vi "BMU参数读取-Auto.vi"(7 "Socket":dbl, 8 "CAN端口":u16(ring), 9 "设备索引号":u16(ring), 10 "CAN卡类型":u32(ring)=21, 11 "从板号":u8=1) -> (3 "成功?":bool)   [LabVIEW 2013] (continued)
                n3264 = Select(t=0, s=w5020, f=1) -> (s? t:f=w5019:i32)
                n3265 = property on="电池组信息" class="Clust (严格)"("Disabled"=w5019) -> ()  [unwired: 2 in, 2 out]
                n3266 = property on="从板号" class="DigNum (严格)"("NumText.BGColor"=u32 16777215) -> ()  [unwired: 2 in, 2 out]
                n3267 = global read "功能码全局.vi" "24"() -> (w5016:bool[])
                n3268 = global read "功能码全局.vi" "23"() -> (w5017:bool[])
                n3269 = Index Array(array=w5016) -> (element #3=w5006:bool, element #4=w5005:bool, element #5=w5004:bool, element #6=w5003:bool, element #7=w5002:bool, element #8=w5001:bool)  [unwired: 8 in, 2 out]
                n3270 = Index Array(array=w5017) -> (element #3=w5015:bool, element #4=w5014:bool, element #5=w5013:bool, element #6=w5012:bool, element #7=w5011:bool, element #8=w5010:bool)  [unwired: 8 in, 2 out]
                n3271 = Build Array(w5006, w5005, w5004, w5003, w5002, w5001) -> (w5007:bool[])
                n3272 = Build Array(w5015, w5014, w5013, w5012, w5011, w5010) -> (w5009:bool[])
                n3273 = And Array Elements(Boolean array=w5007) -> (logical AND=w5000:bool)
                n3274 = And Array Elements(Boolean array=w5009) -> (logical AND=w5008:bool)
                n3275 = Not(x=w4999) -> (.not. x?=w5023:bool)
              }
              frame "电池包信息1" {
                w5028 = 2
                w5036 = 2
                w5027 = 2
                w5025 = FALSE ("1 6")
                n3276 = Select(t=0, s=w5033, f=1) -> (s? t:f=w5026:i32)
                n3277 = property on="串联数" class="DigNum (严格)"("Disabled"=w5026) -> ()  [unwired: 2 in, 2 out]
                n3278 = property on="并联数" class="DigNum (严格)"("Disabled"=w5026) -> ()  [unwired: 2 in, 2 out]
                n3279 = property on="电池厂家" class="DigNum (严格)"("Disabled"=w5026) -> ()  [unwired: 2 in, 2 out]
                n3280 = property on="电池类型" class="DigNum (严格)"("Disabled"=w5026) -> ()  [unwired: 2 in, 2 out]
                n3281 = property on="额定能量" class="DigNum (严格)"("Disabled"=w5026) -> ()  [unwired: 2 in, 2 out]
                n3282 = property on="额定容量" class="DigNum (严格)"("Disabled"=w5026) -> ()  [unwired: 2 in, 2 out]
                n3283 = property on="实际容量" class="DigNum (严格)"("Disabled"=w5026) -> ()  [unwired: 2 in, 2 out]
                n3284 = property on="电池组信息" class="Clust (严格)"("Disabled"=w5026) -> ()  [unwired: 2 in, 2 out]
                n3285 = property on="生产日期" class="Str"("DisabledEnum"=w5026) -> ()  [unwired: 2 in, 2 out]
                n3286 = property on="车牌号" class="Str"("DisabledEnum"=w5027) -> ()  [unwired: 2 in, 2 out]
                n3287 = property on="产权标识" class="DigNum (严格)"("Disabled"=w5026) -> ()  [unwired: 2 in, 2 out]
                n3288 = property on="应用车型" class="DigNum (严格)"("Disabled"=w5026) -> ()  [unwired: 2 in, 2 out]
                n3289 = property on="额定总压" class="DigNum (严格)"("Disabled"=w5026) -> ()  [unwired: 2 in, 2 out]
                n3290 = property on="电池包序号" class="DigNum (严格)"("DisabledEnum"=w5026) -> ()  [unwired: 2 in, 2 out]
                n3291 = property on="电池包组号" class="DigNum (严格)"("DisabledEnum"=w5027) -> ()  [unwired: 2 in, 2 out]
                n3292 = property on="最大允许单体电压" class="DigNum (严格)"("Disabled"=w5036) -> ()  [unwired: 2 in, 2 out]
                n3293 = property on="最大允许总电压" class="DigNum (严格)"("Disabled"=w5036) -> ()  [unwired: 2 in, 2 out]
                n3294 = property on="最大允许温度" class="DigNum (严格)"("Disabled"=w5036) -> ()  [unwired: 2 in, 2 out]
                n3295 = property on="最小允许温度" class="DigNum (严格)"("Disabled"=w5036) -> ()  [unwired: 2 in, 2 out]
                n3296 = property on="最大允许充电电流" class="DigNum (严格)"("Disabled"=w5036) -> ()  [unwired: 2 in, 2 out]
                n3297 = property on="最小允许充电电流" class="DigNum (严格)"("Disabled"=w5036) -> ()  [unwired: 2 in, 2 out]
                n3298 = property on="最小允许单体电压" class="DigNum (严格)"("Disabled"=w5036) -> ()  [unwired: 2 in, 2 out]
                n3299 = property on="电流步长" class="DigNum (严格)"("Disabled"=w5036) -> ()  [unwired: 2 in, 2 out]
                n3300 = property on="SOC" class="DigNum (严格)"("Disabled"=w5036) -> ()  [unwired: 2 in, 2 out]
                n3301 = property on="充电总安时" class="DigNum (严格)"("Disabled"=w5036) -> ()  [unwired: 2 in, 2 out]
                n3302 = property on="放电总安时" class="DigNum (严格)"("Disabled"=w5036) -> ()  [unwired: 2 in, 2 out]
                n3303 = property on="放空次数" class="DigNum (严格)"("DisabledEnum"=w5028) -> ()  [unwired: 2 in, 2 out]
                n3304 = property on="充满次数" class="DigNum (严格)"("DisabledEnum"=w5028) -> ()  [unwired: 2 in, 2 out]
                n3305 = property on="充电次数" class="DigNum (严格)"("DisabledEnum"=w5028) -> ()  [unwired: 2 in, 2 out]
                n3306 = global read "功能码全局.vi" "24"() -> (w5031:bool[])
                n3307 = global read "功能码全局.vi" "23"() -> (w5032:bool[])
                n3308 = Index Array(array=w5031) -> (element #3=w5029:bool)  [unwired: 8 in, 7 out]
                n3309 = Index Array(array=w5032) -> (element #3=w5030:bool)  [unwired: 8 in, 7 out]
                n3310 = Not(x=w5025) -> (.not. x?=w5037:bool)
              }
              frame "电池包组号" {
                w5042 = 2
                w5041 = 2
                w5051 = 2
                w5043 = 2
                w5052 = 2
                w5039 = FALSE ("1 6")
                n3311 = property on="串联数" class="DigNum (严格)"("Disabled"=w5052) -> ()  [unwired: 2 in, 2 out]
                n3312 = property on="并联数" class="DigNum (严格)"("Disabled"=w5052) -> ()  [unwired: 2 in, 2 out]
                n3313 = property on="电池厂家" class="DigNum (严格)"("Disabled"=w5052) -> ()  [unwired: 2 in, 2 out]
                n3314 = property on="电池类型" class="DigNum (严格)"("Disabled"=w5052) -> ()  [unwired: 2 in, 2 out]
                n3315 = property on="额定能量" class="DigNum (严格)"("Disabled"=w5052) -> ()  [unwired: 2 in, 2 out]
                n3316 = property on="额定容量" class="DigNum (严格)"("Disabled"=w5052) -> ()  [unwired: 2 in, 2 out]
                n3317 = property on="实际容量" class="DigNum (严格)"("Disabled"=w5052) -> ()  [unwired: 2 in, 2 out]
                n3318 = Select(t=0, s=w5048, f=1) -> (s? t:f=w5040:i32)
                n3319 = property on="生产日期" class="Str"("DisabledEnum"=w5042) -> ()  [unwired: 2 in, 2 out]
                n3320 = property on="电池包序号" class="DigNum (严格)"("DisabledEnum"=w5042) -> ()  [unwired: 2 in, 2 out]
                n3321 = property on="车牌号" class="Str"("DisabledEnum"=w5042) -> ()  [unwired: 2 in, 2 out]
                n3322 = property on="电池包组号" class="DigNum (严格)"("DisabledEnum"=w5040) -> ()  [unwired: 2 in, 2 out]
                n3323 = property on="电池组信息" class="Clust (严格)"("Disabled"=w5040) -> ()  [unwired: 2 in, 2 out]
                n3324 = property on="产权标识" class="DigNum (严格)"("Disabled"=w5043) -> ()  [unwired: 2 in, 2 out]
                n3325 = property on="应用车型" class="DigNum (严格)"("Disabled"=w5043) -> ()  [unwired: 2 in, 2 out]
                n3326 = property on="额定总压" class="DigNum (严格)"("Disabled"=w5043) -> ()  [unwired: 2 in, 2 out]
                n3327 = property on="放空次数" class="DigNum (严格)"("DisabledEnum"=w5041) -> ()  [unwired: 2 in, 2 out]
                n3328 = property on="充满次数" class="DigNum (严格)"("DisabledEnum"=w5041) -> ()  [unwired: 2 in, 2 out]
                n3329 = property on="充电次数" class="DigNum (严格)"("DisabledEnum"=w5041) -> ()  [unwired: 2 in, 2 out]
                n3330 = property on="最大允许单体电压" class="DigNum (严格)"("Disabled"=w5051) -> ()  [unwired: 2 in, 2 out]
                n3331 = property on="最大允许总电压" class="DigNum (严格)"("Disabled"=w5051) -> ()  [unwired: 2 in, 2 out]
                n3332 = property on="最大允许温度" class="DigNum (严格)"("Disabled"=w5051) -> ()  [unwired: 2 in, 2 out]
                n3333 = property on="最小允许温度" class="DigNum (严格)"("Disabled"=w5051) -> ()  [unwired: 2 in, 2 out]
                n3334 = property on="最大允许充电电流" class="DigNum (严格)"("Disabled"=w5051) -> ()  [unwired: 2 in, 2 out]
                n3335 = property on="最小允许充电电流" class="DigNum (严格)"("Disabled"=w5051) -> ()  [unwired: 2 in, 2 out]
                n3336 = property on="最小允许单体电压" class="DigNum (严格)"("Disabled"=w5051) -> ()  [unwired: 2 in, 2 out]
                n3337 = property on="电流步长" class="DigNum (严格)"("Disabled"=w5051) -> ()  [unwired: 2 in, 2 out]
                n3338 = property on="SOC" class="DigNum (严格)"("Disabled"=w5051) -> ()  [unwired: 2 in, 2 out]
                n3339 = property on="充电总安时" class="DigNum (严格)"("Disabled"=w5051) -> ()  [unwired: 2 in, 2 out]
                n3340 = property on="放电总安时" class="DigNum (严格)"("Disabled"=w5051) -> ()  [unwired: 2 in, 2 out]
                n3341 = global read "功能码全局.vi" "24"() -> (w5046:bool[])
                n3342 = global read "功能码全局.vi" "23"() -> (w5047:bool[])
                n3343 = Index Array(array=w5046) -> (element #3=w5044:bool)  [unwired: 8 in, 7 out]
                n3344 = Index Array(array=w5047) -> (element #3=w5045:bool)  [unwired: 8 in, 7 out]
                n3345 = Not(x=w5039) -> (.not. x?=w5053:bool)
              }
              frame "充放电安时" {
                w5057 = 2
                w5056 = 2
                w5066 = 2
                w5067 = 2
                w5069 = 2
                w5055 = FALSE ("1 6")
                n3346 = property on="串联数" class="DigNum (严格)"("Disabled"=w5069) -> ()  [unwired: 2 in, 2 out]
                n3347 = property on="并联数" class="DigNum (严格)"("Disabled"=w5069) -> ()  [unwired: 2 in, 2 out]
                n3348 = property on="电池厂家" class="DigNum (严格)"("Disabled"=w5069) -> ()  [unwired: 2 in, 2 out]
                n3349 = property on="电池类型" class="DigNum (严格)"("Disabled"=w5069) -> ()  [unwired: 2 in, 2 out]
                n3350 = property on="额定能量" class="DigNum (严格)"("Disabled"=w5069) -> ()  [unwired: 2 in, 2 out]
                n3351 = property on="额定容量" class="DigNum (严格)"("Disabled"=w5069) -> ()  [unwired: 2 in, 2 out]
                n3352 = property on="实际容量" class="DigNum (严格)"("Disabled"=w5069) -> ()  [unwired: 2 in, 2 out]
                n3353 = Select(t=0, s=w5063, f=1) -> (s? t:f=w5062:i32)
                n3354 = property on="生产日期" class="Str"("DisabledEnum"=w5057) -> ()  [unwired: 2 in, 2 out]
                n3355 = property on="电池包序号" class="DigNum (严格)"("DisabledEnum"=w5057) -> ()  [unwired: 2 in, 2 out]
                n3356 = property on="车牌号" class="Str"("DisabledEnum"=w5057) -> ()  [unwired: 2 in, 2 out]
                n3357 = property on="电池包组号" class="DigNum (严格)"("DisabledEnum"=w5057) -> ()  [unwired: 2 in, 2 out]
                n3358 = property on="电池组信息" class="Clust (严格)"("Disabled"=w5062) -> ()  [unwired: 2 in, 2 out]
                n3359 = property on="额定总压" class="DigNum (严格)"("Disabled"=2) -> ()  [unwired: 2 in, 2 out]
                n3360 = property on="产权标识" class="DigNum (严格)"("Disabled"=w5067) -> ()  [unwired: 2 in, 2 out]
                n3361 = property on="应用车型" class="DigNum (严格)"("Disabled"=w5067) -> ()  [unwired: 2 in, 2 out]
                n3362 = property on="放空次数" class="DigNum (严格)"("DisabledEnum"=w5056) -> ()  [unwired: 2 in, 2 out]
                n3363 = property on="充满次数" class="DigNum (严格)"("DisabledEnum"=w5056) -> ()  [unwired: 2 in, 2 out]
                n3364 = property on="充电次数" class="DigNum (严格)"("DisabledEnum"=w5056) -> ()  [unwired: 2 in, 2 out]
                n3365 = property on="最大允许单体电压" class="DigNum (严格)"("Disabled"=w5066) -> ()  [unwired: 2 in, 2 out]
                n3366 = property on="最大允许总电压" class="DigNum (严格)"("Disabled"=w5066) -> ()  [unwired: 2 in, 2 out]
                n3367 = property on="最大允许温度" class="DigNum (严格)"("Disabled"=w5066) -> ()  [unwired: 2 in, 2 out]
                n3368 = property on="最小允许温度" class="DigNum (严格)"("Disabled"=w5066) -> ()  [unwired: 2 in, 2 out]
                n3369 = property on="最大允许充电电流" class="DigNum (严格)"("Disabled"=w5066) -> ()  [unwired: 2 in, 2 out]
                n3370 = property on="最小允许充电电流" class="DigNum (严格)"("Disabled"=w5066) -> ()  [unwired: 2 in, 2 out]
                n3371 = property on="最小允许单体电压" class="DigNum (严格)"("Disabled"=w5066) -> ()  [unwired: 2 in, 2 out]
                n3372 = property on="电流步长" class="DigNum (严格)"("Disabled"=w5066) -> ()  [unwired: 2 in, 2 out]
                n3373 = property on="SOC" class="DigNum (严格)"("Disabled"=w5066) -> ()  [unwired: 2 in, 2 out]
                n3374 = property on="充电总安时" class="DigNum (严格)"("Disabled"=w5062) -> ()  [unwired: 2 in, 2 out]
                n3375 = property on="放电总安时" class="DigNum (严格)"("Disabled"=w5062) -> ()  [unwired: 2 in, 2 out]
                n3376 = Not(x=w5055) -> (.not. x?=w5070:bool)
                n3377 = global read "功能码全局.vi" "24"() -> (w5060:bool[])
                n3378 = global read "功能码全局.vi" "23"() -> (w5061:bool[])
                n3379 = Index Array(array=w5060) -> (element #7=w5058:bool)  [unwired: 8 in, 7 out]
                n3380 = Index Array(array=w5061) -> (element #7=w5059:bool)  [unwired: 8 in, 7 out]
              }
              frame "充电次数" {
                w5075 = 2
                w5084 = 2
                w5085 = 2
                w5076 = 2
                w5086 = 2
                w5072 = FALSE ("1 6")
                n3381 = property on="串联数" class="DigNum (严格)"("Disabled"=w5086) -> ()  [unwired: 2 in, 2 out]
                n3382 = property on="并联数" class="DigNum (严格)"("Disabled"=w5086) -> ()  [unwired: 2 in, 2 out]
                n3383 = property on="电池厂家" class="DigNum (严格)"("Disabled"=w5086) -> ()  [unwired: 2 in, 2 out]
                n3384 = property on="电池类型" class="DigNum (严格)"("Disabled"=w5086) -> ()  [unwired: 2 in, 2 out]
                n3385 = property on="额定能量" class="DigNum (严格)"("Disabled"=w5086) -> ()  [unwired: 2 in, 2 out]
                n3386 = property on="额定容量" class="DigNum (严格)"("Disabled"=w5086) -> ()  [unwired: 2 in, 2 out]
                n3387 = property on="实际容量" class="DigNum (严格)"("Disabled"=w5086) -> ()  [unwired: 2 in, 2 out]
                n3388 = Select(t=0, s=w5081, f=1) -> (s? t:f=w5073:i32)
                n3389 = property on="生产日期" class="Str"("DisabledEnum"=w5075) -> ()  [unwired: 2 in, 2 out]
                n3390 = property on="电池包序号" class="DigNum (严格)"("DisabledEnum"=w5075) -> ()  [unwired: 2 in, 2 out]
                n3391 = property on="车牌号" class="Str"("DisabledEnum"=w5075) -> ()  [unwired: 2 in, 2 out]
                n3392 = property on="电池组信息" class="Clust (严格)"("Disabled"=w5073) -> ()  [unwired: 2 in, 2 out]
                n3393 = property on="电池包组号" class="DigNum (严格)"("DisabledEnum"=w5075) -> ()  [unwired: 2 in, 2 out]
                n3394 = property on="额定总压" class="DigNum (严格)"("Disabled"=w5076) -> ()  [unwired: 2 in, 2 out]
                n3395 = property on="产权标识" class="DigNum (严格)"("Disabled"=w5076) -> ()  [unwired: 2 in, 2 out]
                n3396 = property on="应用车型" class="DigNum (严格)"("Disabled"=w5076) -> ()  [unwired: 2 in, 2 out]
                n3397 = property on="放空次数" class="DigNum (严格)"("DisabledEnum"=w5073) -> (error out=w5074:errorcluster)  [unwired: 2 in, 1 out]
                n3398 = property on="充满次数" class="DigNum (严格)"("DisabledEnum"=w5073) -> ()  [unwired: 2 in, 2 out]
                n3399 = property on="充电次数" class="DigNum (严格)"("DisabledEnum"=w5073) -> ()  [unwired: 2 in, 2 out]
                n3400 = property on="最大允许单体电压" class="DigNum (严格)"("Disabled"=w5085) -> ()  [unwired: 2 in, 2 out]
                n3401 = property on="最大允许总电压" class="DigNum (严格)"("Disabled"=w5085) -> ()  [unwired: 2 in, 2 out]
                n3402 = property on="最大允许温度" class="DigNum (严格)"("Disabled"=w5085) -> ()  [unwired: 2 in, 2 out]
                n3403 = property on="最小允许温度" class="DigNum (严格)"("Disabled"=w5085) -> ()  [unwired: 2 in, 2 out]
                n3404 = property on="最大允许充电电流" class="DigNum (严格)"("Disabled"=w5085) -> ()  [unwired: 2 in, 2 out]
                n3405 = property on="最小允许充电电流" class="DigNum (严格)"(error in=w5074, "Disabled"=w5085) -> ()  [unwired: 1 in, 2 out]
                n3406 = property on="最小允许单体电压" class="DigNum (严格)"("Disabled"=w5085) -> ()  [unwired: 2 in, 2 out]
                n3407 = property on="电流步长" class="DigNum (严格)"("Disabled"=w5085) -> ()  [unwired: 2 in, 2 out]
                n3408 = property on="SOC" class="DigNum (严格)"("Disabled"=w5085) -> ()  [unwired: 2 in, 2 out]
                n3409 = property on="充电总安时" class="DigNum (严格)"("Disabled"=w5084) -> ()  [unwired: 2 in, 2 out]
                n3410 = property on="放电总安时" class="DigNum (严格)"("Disabled"=w5084) -> ()  [unwired: 2 in, 2 out]
                n3411 = Not(x=w5072) -> (.not. x?=w5087:bool)
                n3412 = global read "功能码全局.vi" "24"() -> (w5079:bool[])
                n3413 = global read "功能码全局.vi" "23"() -> (w5080:bool[])
                n3414 = Index Array(array=w5079) -> (element #8=w5078:bool)  [unwired: 8 in, 7 out]
                n3415 = Index Array(array=w5080) -> (element #8=w5077:bool)  [unwired: 8 in, 7 out]
              }
              frame "SOC" {
                w5091 = 2
                w5090 = 2
                w5100 = 2
                w5101 = 2
                w5102 = 2
                w5104 = 2
                w5089 = FALSE ("1 6")
                n3416 = property on="串联数" class="DigNum (严格)"("Disabled"=w5104) -> ()  [unwired: 2 in, 2 out]
                n3417 = property on="并联数" class="DigNum (严格)"("Disabled"=w5104) -> ()  [unwired: 2 in, 2 out]
                n3418 = property on="电池厂家" class="DigNum (严格)"("Disabled"=w5104) -> ()  [unwired: 2 in, 2 out]
                n3419 = property on="电池类型" class="DigNum (严格)"("Disabled"=w5104) -> ()  [unwired: 2 in, 2 out]
                n3420 = property on="额定能量" class="DigNum (严格)"("Disabled"=w5104) -> ()  [unwired: 2 in, 2 out]
                n3421 = property on="额定容量" class="DigNum (严格)"("Disabled"=w5104) -> ()  [unwired: 2 in, 2 out]
                n3422 = property on="实际容量" class="DigNum (严格)"("Disabled"=w5104) -> ()  [unwired: 2 in, 2 out]
                n3423 = Select(t=0, s=w5097, f=1) -> (s? t:f=w5096:i32)
                n3424 = property on="生产日期" class="Str"("DisabledEnum"=w5091) -> ()  [unwired: 2 in, 2 out]
                n3425 = property on="电池包序号" class="DigNum (严格)"("DisabledEnum"=w5091) -> ()  [unwired: 2 in, 2 out]
                n3426 = property on="车牌号" class="Str"("DisabledEnum"=w5091) -> ()  [unwired: 2 in, 2 out]
                n3427 = property on="电池包组号" class="DigNum (严格)"("DisabledEnum"=w5091) -> ()  [unwired: 2 in, 2 out]
                n3428 = property on="电池组信息" class="Clust (严格)"("Disabled"=w5096) -> ()  [unwired: 2 in, 2 out]
                n3429 = property on="SOC" class="DigNum (严格)"("Disabled"=w5096) -> ()  [unwired: 2 in, 2 out]
                n3430 = property on="额定总压" class="DigNum (严格)"("Disabled"=2) -> ()  [unwired: 2 in, 2 out]
                n3431 = property on="产权标识" class="DigNum (严格)"("Disabled"=w5102) -> ()  [unwired: 2 in, 2 out]
                n3432 = property on="应用车型" class="DigNum (严格)"("Disabled"=w5102) -> ()  [unwired: 2 in, 2 out]
                n3433 = property on="放空次数" class="DigNum (严格)"("DisabledEnum"=w5090) -> ()  [unwired: 2 in, 2 out]
                n3434 = property on="充满次数" class="DigNum (严格)"("DisabledEnum"=w5090) -> ()  [unwired: 2 in, 2 out]
                n3435 = property on="充电次数" class="DigNum (严格)"("DisabledEnum"=w5090) -> ()  [unwired: 2 in, 2 out]
                n3436 = property on="最大允许单体电压" class="DigNum (严格)"("Disabled"=w5101) -> ()  [unwired: 2 in, 2 out]
                n3437 = property on="最大允许总电压" class="DigNum (严格)"("Disabled"=w5101) -> ()  [unwired: 2 in, 2 out]
                n3438 = property on="最大允许温度" class="DigNum (严格)"("Disabled"=w5101) -> ()  [unwired: 2 in, 2 out]
                n3439 = property on="最小允许温度" class="DigNum (严格)"("Disabled"=w5101) -> ()  [unwired: 2 in, 2 out]
                n3440 = property on="最大允许充电电流" class="DigNum (严格)"("Disabled"=w5101) -> ()  [unwired: 2 in, 2 out]
                n3441 = property on="最小允许充电电流" class="DigNum (严格)"("Disabled"=w5101) -> ()  [unwired: 2 in, 2 out]
                n3442 = property on="最小允许单体电压" class="DigNum (严格)"("Disabled"=w5101) -> ()  [unwired: 2 in, 2 out]
                n3443 = property on="电流步长" class="DigNum (严格)"("Disabled"=w5101) -> ()  [unwired: 2 in, 2 out]
                n3444 = property on="充电总安时" class="DigNum (严格)"("Disabled"=w5100) -> ()  [unwired: 2 in, 2 out]
                n3445 = property on="放电总安时" class="DigNum (严格)"("Disabled"=w5100) -> ()  [unwired: 2 in, 2 out]
                n3446 = Not(x=w5089) -> (.not. x?=w5105:bool)
                n3447 = global read "功能码全局.vi" "24"() -> (w5094:bool[])
                n3448 = global read "功能码全局.vi" "23"() -> (w5095:bool[])
                n3449 = Index Array(array=w5094) -> (element #6=w5093:bool)  [unwired: 8 in, 7 out]
                n3450 = Index Array(array=w5095) -> (element #6=w5092:bool)  [unwired: 8 in, 7 out]
              }
              frame "车牌号" {
                w5110 = 2
                w5109 = 2
                w5119 = 2
                w5120 = 2
                w5121 = 2
                w5123 = 2
                w5107 = FALSE ("1 6")
                n3451 = property on="串联数" class="DigNum (严格)"("Disabled"=w5123) -> ()  [unwired: 2 in, 2 out]
                n3452 = property on="并联数" class="DigNum (严格)"("Disabled"=w5123) -> ()  [unwired: 2 in, 2 out]
                n3453 = property on="电池厂家" class="DigNum (严格)"("Disabled"=w5123) -> ()  [unwired: 2 in, 2 out]
                n3454 = property on="电池类型" class="DigNum (严格)"("Disabled"=w5123) -> ()  [unwired: 2 in, 2 out]
                n3455 = property on="额定能量" class="DigNum (严格)"("Disabled"=w5123) -> ()  [unwired: 2 in, 2 out]
                n3456 = property on="额定容量" class="DigNum (严格)"("Disabled"=w5123) -> ()  [unwired: 2 in, 2 out]
                n3457 = property on="实际容量" class="DigNum (严格)"("Disabled"=w5123) -> ()  [unwired: 2 in, 2 out]
                n3458 = Select(t=0, s=w5115, f=1) -> (s? t:f=w5108:i32)
                n3459 = property on="生产日期" class="Str"("DisabledEnum"=w5110) -> ()  [unwired: 2 in, 2 out]
                n3460 = property on="电池包序号" class="DigNum (严格)"("DisabledEnum"=w5110) -> ()  [unwired: 2 in, 2 out]
                n3461 = property on="电池包组号" class="DigNum (严格)"("DisabledEnum"=w5110) -> ()  [unwired: 2 in, 2 out]
                n3462 = property on="电池组信息" class="Clust (严格)"("Disabled"=w5108) -> ()  [unwired: 2 in, 2 out]
                n3463 = property on="车牌号" class="Str"("DisabledEnum"=w5108) -> ()  [unwired: 2 in, 2 out]
                n3464 = property on="额定总压" class="DigNum (严格)"("Disabled"=2) -> ()  [unwired: 2 in, 2 out]
                n3465 = property on="产权标识" class="DigNum (严格)"("Disabled"=w5121) -> ()  [unwired: 2 in, 2 out]
                n3466 = property on="应用车型" class="DigNum (严格)"("Disabled"=w5121) -> ()  [unwired: 2 in, 2 out]
                n3467 = property on="放空次数" class="DigNum (严格)"("DisabledEnum"=w5109) -> ()  [unwired: 2 in, 2 out]
                n3468 = property on="充满次数" class="DigNum (严格)"("DisabledEnum"=w5109) -> ()  [unwired: 2 in, 2 out]
                n3469 = property on="充电次数" class="DigNum (严格)"("DisabledEnum"=w5109) -> ()  [unwired: 2 in, 2 out]
                n3470 = property on="最大允许单体电压" class="DigNum (严格)"("Disabled"=w5120) -> ()  [unwired: 2 in, 2 out]
                n3471 = property on="最大允许总电压" class="DigNum (严格)"("Disabled"=w5120) -> ()  [unwired: 2 in, 2 out]
                n3472 = property on="最大允许温度" class="DigNum (严格)"("Disabled"=w5120) -> ()  [unwired: 2 in, 2 out]
                n3473 = property on="最小允许温度" class="DigNum (严格)"("Disabled"=w5120) -> ()  [unwired: 2 in, 2 out]
                n3474 = property on="最大允许充电电流" class="DigNum (严格)"("Disabled"=w5120) -> ()  [unwired: 2 in, 2 out]
                n3475 = property on="最小允许充电电流" class="DigNum (严格)"("Disabled"=w5120) -> ()  [unwired: 2 in, 2 out]
                n3476 = property on="最小允许单体电压" class="DigNum (严格)"("Disabled"=w5120) -> ()  [unwired: 2 in, 2 out]
                n3477 = property on="电流步长" class="DigNum (严格)"("Disabled"=w5120) -> ()  [unwired: 2 in, 2 out]
                n3478 = property on="SOC" class="DigNum (严格)"("Disabled"=2) -> ()  [unwired: 2 in, 2 out]
                n3479 = property on="充电总安时" class="DigNum (严格)"("Disabled"=w5119) -> ()  [unwired: 2 in, 2 out]
                n3480 = property on="放电总安时" class="DigNum (严格)"("Disabled"=w5119) -> ()  [unwired: 2 in, 2 out]
                n3481 = Not(x=w5107) -> (.not. x?=w5124:bool)
                n3482 = global read "功能码全局.vi" "24"() -> (w5113:bool[])
                n3483 = global read "功能码全局.vi" "23"() -> (w5114:bool[])
                n3484 = Index Array(array=w5113) -> (element #5=w5111:bool)  [unwired: 8 in, 7 out]
                n3485 = Index Array(array=w5114) -> (element #5=w5112:bool)  [unwired: 8 in, 7 out]
              }
              frame "充电参数" {
                w5128 = 2
                w5127 = 2
                w5137 = 2
                w5138 = 2
                w5140 = 2
                w5126 = FALSE ("1 6")
                n3486 = property on="串联数" class="DigNum (严格)"("Disabled"=w5140) -> ()  [unwired: 2 in, 2 out]
                n3487 = property on="并联数" class="DigNum (严格)"("Disabled"=w5140) -> ()  [unwired: 2 in, 2 out]
                n3488 = property on="电池厂家" class="DigNum (严格)"("Disabled"=w5140) -> ()  [unwired: 2 in, 2 out]
                n3489 = property on="电池类型" class="DigNum (严格)"("Disabled"=w5140) -> ()  [unwired: 2 in, 2 out]
                n3490 = property on="额定能量" class="DigNum (严格)"("Disabled"=w5140) -> ()  [unwired: 2 in, 2 out]
                n3491 = property on="额定容量" class="DigNum (严格)"("Disabled"=w5140) -> ()  [unwired: 2 in, 2 out]
                n3492 = property on="实际容量" class="DigNum (严格)"("Disabled"=w5140) -> ()  [unwired: 2 in, 2 out]
                n3493 = Select(t=0, s=w5134, f=1) -> (s? t:f=w5133:i32)
                n3494 = property on="生产日期" class="Str"("DisabledEnum"=w5128) -> ()  [unwired: 2 in, 2 out]
                n3495 = property on="电池包序号" class="DigNum (严格)"("DisabledEnum"=w5128) -> ()  [unwired: 2 in, 2 out]
                n3496 = property on="车牌号" class="Str"("DisabledEnum"=w5128) -> ()  [unwired: 2 in, 2 out]
                n3497 = property on="电池组信息" class="Clust (严格)"("Disabled"=w5133) -> ()  [unwired: 2 in, 2 out]
                n3498 = property on="电池包组号" class="DigNum (严格)"("DisabledEnum"=w5128) -> ()  [unwired: 2 in, 2 out]
                n3499 = property on="额定总压" class="DigNum (严格)"("Disabled"=2) -> ()  [unwired: 2 in, 2 out]
                n3500 = property on="产权标识" class="DigNum (严格)"("Disabled"=w5138) -> ()  [unwired: 2 in, 2 out]
                n3501 = property on="应用车型" class="DigNum (严格)"("Disabled"=w5138) -> ()  [unwired: 2 in, 2 out]
                n3502 = property on="放空次数" class="DigNum (严格)"("DisabledEnum"=w5127) -> ()  [unwired: 2 in, 2 out]
                n3503 = property on="充满次数" class="DigNum (严格)"("DisabledEnum"=w5127) -> ()  [unwired: 2 in, 2 out]
                n3504 = property on="充电次数" class="DigNum (严格)"("DisabledEnum"=w5127) -> ()  [unwired: 2 in, 2 out]
                n3505 = property on="最大允许单体电压" class="DigNum (严格)"("Disabled"=w5133) -> ()  [unwired: 2 in, 2 out]
                n3506 = property on="最大允许总电压" class="DigNum (严格)"("Disabled"=w5133) -> ()  [unwired: 2 in, 2 out]
                n3507 = property on="最大允许温度" class="DigNum (严格)"("Disabled"=w5133) -> ()  [unwired: 2 in, 2 out]
                n3508 = property on="最小允许温度" class="DigNum (严格)"("Disabled"=w5133) -> ()  [unwired: 2 in, 2 out]
                n3509 = property on="最大允许充电电流" class="DigNum (严格)"("Disabled"=w5133) -> ()  [unwired: 2 in, 2 out]
                n3510 = property on="最小允许充电电流" class="DigNum (严格)"("Disabled"=w5133) -> ()  [unwired: 2 in, 2 out]
                n3511 = property on="最小允许单体电压" class="DigNum (严格)"("Disabled"=w5133) -> ()  [unwired: 2 in, 2 out]
                n3512 = property on="电流步长" class="DigNum (严格)"("Disabled"=w5133) -> ()  [unwired: 2 in, 2 out]
                n3513 = property on="SOC" class="DigNum (严格)"("Disabled"=w5137) -> ()  [unwired: 2 in, 2 out]
                n3514 = property on="充电总安时" class="DigNum (严格)"("Disabled"=w5137) -> ()  [unwired: 2 in, 2 out]
                n3515 = property on="放电总安时" class="DigNum (严格)"("Disabled"=w5137) -> ()  [unwired: 2 in, 2 out]
                n3516 = Not(x=w5126) -> (.not. x?=w5141:bool)
                n3517 = global read "功能码全局.vi" "24"() -> (w5131:bool[])
                n3518 = global read "功能码全局.vi" "23"() -> (w5132:bool[])
                n3519 = Index Array(array=w5131) -> (element #4=w5129:bool)  [unwired: 8 in, 7 out]
                n3520 = Index Array(array=w5132) -> (element #4=w5130:bool)  [unwired: 8 in, 7 out]
              }
              frame "均衡参数" {
                w5143 = FALSE ("1 6")
                n3521 = Select(t=0, s=w5149, f=1) -> (s? t:f=w5147:i32)
                n3522 = property on="均衡计算-电压高阀值1级" class="DigNum (严格)"("DisabledEnum"=w5147) -> ()  [unwired: 2 in, 2 out]
                n3523 = property on="均衡计算-电压高阀值2级" class="DigNum (严格)"("DisabledEnum"=w5147) -> ()  [unwired: 2 in, 2 out]
                n3524 = property on="均衡计算-电压低阀值1级" class="DigNum (严格)"("DisabledEnum"=w5147) -> ()  [unwired: 2 in, 2 out]
                n3525 = property on="均衡计算-电压低阀值2级" class="DigNum (严格)"("DisabledEnum"=w5147) -> ()  [unwired: 2 in, 2 out]
                n3526 = property on="均衡计算-最低电压阀值" class="DigNum (严格)"("DisabledEnum"=w5147) -> ()  [unwired: 2 in, 2 out]
                n3527 = property on="均衡停止-最低电压阀值" class="DigNum (严格)"("DisabledEnum"=w5147) -> ()  [unwired: 2 in, 2 out]
                n3528 = property on="均衡计算-电压极差阀值" class="DigNum (严格)"("DisabledEnum"=w5147) -> ()  [unwired: 2 in, 2 out]
                n3529 = property on="均衡参数" class="Clust (严格)"("DisabledEnum"=w5147) -> ()  [unwired: 2 in, 2 out]
                n3530 = property on="充电结束电压(90%)" class="DigNum (严格)"("DisabledEnum"=w5147) -> ()  [unwired: 2 in, 2 out]
                n3531 = property on="充电结束电压(91%)" class="DigNum (严格)"("DisabledEnum"=w5147) -> ()  [unwired: 2 in, 2 out]
                n3532 = property on="充电结束电压(92%)" class="DigNum (严格)"("DisabledEnum"=w5147) -> ()  [unwired: 2 in, 2 out]
                n3533 = property on="充电结束电压(93%)" class="DigNum (严格)"("DisabledEnum"=w5147) -> ()  [unwired: 2 in, 2 out]
                n3534 = property on="充电结束电压(94%)" class="DigNum (严格)"("DisabledEnum"=w5147) -> ()  [unwired: 2 in, 2 out]
                n3535 = property on="充电结束电压(95%)" class="DigNum (严格)"("DisabledEnum"=w5147) -> ()  [unwired: 2 in, 2 out]
                n3536 = property on="充电结束电压(96%)" class="DigNum (严格)"("DisabledEnum"=w5147) -> ()  [unwired: 2 in, 2 out]
                n3537 = property on="充电结束电压(97%)" class="DigNum (严格)"("DisabledEnum"=w5147) -> ()  [unwired: 2 in, 2 out]
                n3538 = property on="充电结束电压(98%)" class="DigNum (严格)"("DisabledEnum"=w5147) -> ()  [unwired: 2 in, 2 out]
                n3539 = property on="充电结束电压(99%)" class="DigNum (严格)"("DisabledEnum"=w5147) -> ()  [unwired: 2 in, 2 out]
                n3540 = property on="充电结束电压(100%)" class="DigNum (严格)"("DisabledEnum"=w5147) -> ()  [unwired: 2 in, 2 out]
                n3541 = disable-structure shown="启用" {
                  disable-tunnel: [w5153 w5155] -> w5146
                  disable-tunnel: [w5152 w5155] -> w5145
                  frame Enabled {
                    n3542 = global read "功能码全局.vi" "18"() -> (w5154:bool[])
                    n3543 = Index Array(array=w5154) -> (element #1=w5153:bool, element #2=w5152:bool)  [unwired: 8 in, 6 out]
                  }
                  frame Disabled {
                    w5155 = TRUE
                  }
                }
                n3544 = Not(x=w5143) -> (.not. x?=w5144:bool)
              }
              frame "均衡阀值" {
                w5158 = 2
                w5156 = FALSE ("1 6")
                n3545 = Select(t=0, s=w5163, f=1) -> (s? t:f=w5161:i32)
                n3546 = property on="均衡计算-电压高阀值1级" class="DigNum (严格)"("DisabledEnum"=w5161) -> ()  [unwired: 2 in, 2 out]
                n3547 = property on="均衡计算-电压高阀值2级" class="DigNum (严格)"("DisabledEnum"=w5161) -> ()  [unwired: 2 in, 2 out]
                n3548 = property on="均衡计算-电压低阀值1级" class="DigNum (严格)"("DisabledEnum"=w5161) -> ()  [unwired: 2 in, 2 out]
                n3549 = property on="均衡计算-电压低阀值2级" class="DigNum (严格)"("DisabledEnum"=w5161) -> ()  [unwired: 2 in, 2 out]
                n3550 = property on="均衡计算-最低电压阀值" class="DigNum (严格)"("DisabledEnum"=w5161) -> ()  [unwired: 2 in, 2 out]
                n3551 = property on="均衡停止-最低电压阀值" class="DigNum (严格)"("DisabledEnum"=w5161) -> ()  [unwired: 2 in, 2 out]
                n3552 = property on="均衡计算-电压极差阀值" class="DigNum (严格)"("DisabledEnum"=w5161) -> ()  [unwired: 2 in, 2 out]
                n3553 = property on="均衡参数" class="Clust (严格)"("DisabledEnum"=w5161) -> ()  [unwired: 2 in, 2 out]
                n3554 = property on="充电结束电压(90%)" class="DigNum (严格)"("DisabledEnum"=w5158) -> ()  [unwired: 2 in, 2 out]
                n3555 = property on="充电结束电压(91%)" class="DigNum (严格)"("DisabledEnum"=w5158) -> ()  [unwired: 2 in, 2 out]
                n3556 = property on="充电结束电压(92%)" class="DigNum (严格)"("DisabledEnum"=w5158) -> ()  [unwired: 2 in, 2 out]
                n3557 = property on="充电结束电压(93%)" class="DigNum (严格)"("DisabledEnum"=w5158) -> ()  [unwired: 2 in, 2 out]
                n3558 = property on="充电结束电压(94%)" class="DigNum (严格)"("DisabledEnum"=w5158) -> ()  [unwired: 2 in, 2 out]
                n3559 = property on="充电结束电压(95%)" class="DigNum (严格)"("DisabledEnum"=w5158) -> ()  [unwired: 2 in, 2 out]
                n3560 = property on="充电结束电压(96%)" class="DigNum (严格)"("DisabledEnum"=w5158) -> ()  [unwired: 2 in, 2 out]
                n3561 = property on="充电结束电压(97%)" class="DigNum (严格)"("DisabledEnum"=w5158) -> ()  [unwired: 2 in, 2 out]
                n3562 = property on="充电结束电压(98%)" class="DigNum (严格)"("DisabledEnum"=w5158) -> ()  [unwired: 2 in, 2 out]
                n3563 = property on="充电结束电压(99%)" class="DigNum (严格)"("DisabledEnum"=w5158) -> ()  [unwired: 2 in, 2 out]
                n3564 = property on="充电结束电压(100%)" class="DigNum (严格)"("DisabledEnum"=w5158) -> ()  [unwired: 2 in, 2 out]
                n3565 = disable-structure shown="启用" {
                  disable-tunnel: [w5167 w5169] -> w5160
                  disable-tunnel: [w5166 w5169] -> w5159
                  frame Enabled {
                    n3566 = global read "功能码全局.vi" "18"() -> (w5168:bool[])
                    n3567 = Index Array(array=w5168) -> (element #1=w5167:bool, element #2=w5166:bool)  [unwired: 8 in, 6 out]
                  }
                  frame Disabled {
                    w5169 = TRUE
                  }
                }
                n3568 = Not(x=w5156) -> (.not. x?=w5157:bool)
              }
              frame "充电结束电压" {
                w5173 = 2
                w5170 = FALSE ("1 6")
                n3569 = Select(t=0, s=w5177, f=1) -> (s? t:f=w5172:i32)
                n3570 = property on="均衡计算-电压高阀值1级" class="DigNum (严格)"("DisabledEnum"=w5173) -> ()  [unwired: 2 in, 2 out]
                n3571 = property on="均衡计算-电压高阀值2级" class="DigNum (严格)"("DisabledEnum"=w5173) -> ()  [unwired: 2 in, 2 out]
                n3572 = property on="均衡计算-电压低阀值1级" class="DigNum (严格)"("DisabledEnum"=w5173) -> ()  [unwired: 2 in, 2 out]
                n3573 = property on="均衡计算-电压低阀值2级" class="DigNum (严格)"("DisabledEnum"=w5173) -> ()  [unwired: 2 in, 2 out]
                n3574 = property on="均衡计算-最低电压阀值" class="DigNum (严格)"("DisabledEnum"=w5173) -> ()  [unwired: 2 in, 2 out]
                n3575 = property on="均衡停止-最低电压阀值" class="DigNum (严格)"("DisabledEnum"=w5173) -> ()  [unwired: 2 in, 2 out]
                n3576 = property on="均衡计算-电压极差阀值" class="DigNum (严格)"("DisabledEnum"=w5173) -> ()  [unwired: 2 in, 2 out]
                n3577 = property on="均衡参数" class="Clust (严格)"("DisabledEnum"=w5172) -> ()  [unwired: 2 in, 2 out]
                n3578 = property on="充电结束电压(90%)" class="DigNum (严格)"("DisabledEnum"=w5172) -> ()  [unwired: 2 in, 2 out]
                n3579 = property on="充电结束电压(91%)" class="DigNum (严格)"("DisabledEnum"=w5172) -> ()  [unwired: 2 in, 2 out]
                n3580 = property on="充电结束电压(92%)" class="DigNum (严格)"("DisabledEnum"=w5172) -> ()  [unwired: 2 in, 2 out]
                n3581 = property on="充电结束电压(93%)" class="DigNum (严格)"("DisabledEnum"=w5172) -> ()  [unwired: 2 in, 2 out]
                n3582 = property on="充电结束电压(94%)" class="DigNum (严格)"("DisabledEnum"=w5172) -> ()  [unwired: 2 in, 2 out]
                n3583 = property on="充电结束电压(95%)" class="DigNum (严格)"("DisabledEnum"=w5172) -> ()  [unwired: 2 in, 2 out]
                n3584 = property on="充电结束电压(96%)" class="DigNum (严格)"("DisabledEnum"=w5172) -> ()  [unwired: 2 in, 2 out]
                n3585 = property on="充电结束电压(97%)" class="DigNum (严格)"("DisabledEnum"=w5172) -> ()  [unwired: 2 in, 2 out]
                n3586 = property on="充电结束电压(98%)" class="DigNum (严格)"("DisabledEnum"=w5172) -> ()  [unwired: 2 in, 2 out]
                n3587 = property on="充电结束电压(99%)" class="DigNum (严格)"("DisabledEnum"=w5172) -> ()  [unwired: 2 in, 2 out]
                n3588 = property on="充电结束电压(100%)" class="DigNum (严格)"("DisabledEnum"=w5172) -> ()  [unwired: 2 in, 2 out]
                n3589 = disable-structure shown="启用" {
                  disable-tunnel: [w5181 w5183] -> w5175
                  disable-tunnel: [w5180 w5183] -> w5174
                  frame Enabled {
                    n3590 = global read "功能码全局.vi" "18"() -> (w5182:bool[])
                    n3591 = Index Array(array=w5182) -> (element #1=w5181:bool, element #2=w5180:bool)  [unwired: 8 in, 6 out]
                  }
                  frame Disabled {
                    w5183 = TRUE
                  }
                }
                n3592 = Not(x=w5170) -> (.not. x?=w5171:bool)
              }
              frame "假", Default {
                w5184 = FALSE ("1 6")
                n3593 = Not(x=w5184) -> (.not. x?=w5185:bool)
              }
            }
            n3594 = local write "等级 2"(w4765) -> ()
            n3595 = local write "1 6"(w4764) -> ()
            n3596 = local write "1 7"(w4763) -> ()
            n3597 = local write "1 8"(w4762) -> ()
            n3598 = local write "1 9"(w4761) -> ()
            n3599 = local write "1 10"(w4760) -> ()
            n3600 = local write "1 12"(w4754) -> ()
            n3601 = property on="单个读取" class="Bool (严格)"("Visible"=w4759) -> ()  [unwired: 2 in, 2 out]
            n3602 = property on="单个写入" class="Bool (严格)"("Visible"=w4758) -> ()  [unwired: 2 in, 2 out]
          }
          event "从板个数": Value Change {
            n3603 = event-data() -> ()  [unwired: 7 out]
            n3604 = local read "从板个数"() -> (w5187:dbl)
            n3605 = call "多从板对应参数-new.vi"("从板个数"=w5187) -> ("输出数组"=w5188:string[])  [unwired: 1 in]
            n3606 = control-ref of="项目信息"() -> (w5189:refnum<vi>)
            n3607 = stacked-sequence {
              tunnel: w5189 -> [_ w5196 w5200]
              tunnel: w5188 -> [_ w5195 w5199]
              frame #0 {
                n3608 = local write "项目信息"(string[][] [] ("项目信息")) -> ()
              }
              frame #1 {
                n3609 = call "表格数据输入-8.6.vi"("行数"=u32 0, "列数"=u32 0, "字符串数组"=w5195, "表格引用"=w5196) -> ()  [unwired: 8 out]
              }
              frame #2 {
                n3610 = Array Size(array=w5199) -> (size(s)=w5198:i32)
                n3611 = for {
                  N: w5198 -> [_]
                  tunnel: [""] -> w5197 mode=indexing
                }
                n3612 = call "表格数据输入-8.6.vi"("行数"=u32 0, "列数"=u32 1, "字符串数组"=w5197, "表格引用"=w5200) -> ()  [unwired: 8 out]
              }
            }
          }
          event "主界面选项": Value Change {
            n3613 = event-data() -> ("NewVal"=w5204:enum32{"单选选项1", "单选选项2", "单选选项2 2", "单选选项2 3"})  [unwired: 6 out]
            n3614 = control-ref of="单选选项2 2"() -> (w5209:refnum<vi>)
            n3615 = control-ref of="单选选项2"() -> (w5211:refnum<vi>)
            n3616 = control-ref of="单选选项1"() -> (w5210:refnum<vi>)
            n3617 = control-ref of="单选选项2 3"() -> (w5205:refnum<vi>)
            n3618 = Build Array(w5210, w5211, w5209, w5205) -> (w5208:refnum<vi>[])
            n3619 = case shown="\"单选选项2 2\"" w5204 {
              selector: w5204 -> [w5222 w5227 w5232 w5237]
              tunnel: w5208 -> [w5223 w5228 w5233 w5238]
              tunnel: [w5221 w5226 w5231 w5236] -> w5214
              tunnel: [w5220 w5225 w5230 w5235] -> w5213
              tunnel: [enum32{"读写参数", "版本读取", "其它诊断"}."读写参数" ("选项卡控件 2") enum32{"读写参数", "版本读取", "其它诊断"}."版本读取" ("选项卡控件 2") enum32{"读写参数", "版本读取", "其它诊断"}."其它诊断" ("选项卡控件 2") enum32{"读写参数", "版本读取", "其它诊断", "高压板校正"}."高压板校正" ("选项卡控件 2")] -> w5212
              frame "单选选项1", Default {
                n3620 = Delete From Array(array=w5223, index=w5222) -> (deleted portion=w5220:refnum<vi>, array with subset deleted=w5221:refnum<vi>[])  [unwired: 1 in]
              }
              frame "单选选项2" {
                n3621 = Delete From Array(array=w5228, index=w5227) -> (deleted portion=w5225:refnum<vi>, array with subset deleted=w5226:refnum<vi>[])  [unwired: 1 in]
              }
              frame "单选选项2 2" {
                n3622 = Delete From Array(array=w5233, index=w5232) -> (deleted portion=w5230:refnum<vi>, array with subset deleted=w5231:refnum<vi>[])  [unwired: 1 in]
              }
              frame "单选选项2 3" {
                n3623 = Delete From Array(array=w5238, index=w5237) -> (deleted portion=w5235:refnum<vi>, array with subset deleted=w5236:refnum<vi>[])  [unwired: 1 in]
              }
            }
            n3624 = local write "面板选择"(w5212) -> ()
            n3625 = for {
              tunnel: u32 16777215 -> [w5218]
              tunnel: w5214 -> [w5217] mode=indexing
              n3626 = property class="Bool (严格)"(reference=w5217, "BoolText.TextColor"=w5218) -> ()  [unwired: 1 in, 2 out]
            }
            n3627 = property class="Bool (严格)"(reference=w5213, "BoolText.TextColor"=u32 65511) -> ()  [unwired: 1 in, 2 out]
          }
          event "主从板": Value Change {
            w5240 = FALSE ("可见")
            n3628 = event-data() -> ()  [unwired: 7 out]
            n3629 = control-ref of="单选选项2"() -> (w5248:refnum<vi>)
            n3630 = control-ref of="单选选项1"() -> (w5247:refnum<vi>)
            n3631 = local read "主从板"() -> (w5255:enum32{"单选选项2", "单选选项1"})
            n3632 = Build Array(w5248, w5247) -> (w5254:refnum<vi>[])
            n3633 = case shown="\"单选选项2\"" w5255 {
              selector: w5255 -> [w5300 w5343]
              tunnel: w5254 -> [w5301 w5342]
              tunnel: [enum32{"主板", "从板"}."主板" ("主从选择") enum32{"主板", "从板"}."从板" ("主从选择")] -> w5253
              tunnel: [w5299 w5341] -> w5250
              tunnel: [w5298 w5340] -> w5249
              tunnel: [TRUE FALSE] -> w5245
              tunnel: [w5259 w5320] -> w5242
              tunnel: [w5260 w5325] -> w5241
              tunnel: [FALSE ("可见") TRUE ("可见")] -> w5239
              frame "单选选项1", Default {
                n3634 = global read "功能码全局.vi" "主板项目信息7"() -> (w5271:bool[])
                n3635 = global read "功能码全局.vi" "主板项目信息4"() -> (w5294:bool[])
                n3636 = global read "功能码全局.vi" "主板控制类信息10"() -> (w5275:bool[])
                n3637 = global read "功能码全局.vi" "主板故障阀值9"() -> (w5272:bool[])
                n3638 = global read "功能码全局.vi" "主板项目信息5"() -> (w5285:bool[])
                n3639 = global read "功能码全局.vi" "主板项目信息6"() -> (w5295:bool[])
                n3640 = global read "功能码全局.vi" "主板版本号11"() -> (w5286:bool[])
                n3641 = Delete From Array(array=w5295, length=1 ("长度"), index=0 ("索引")) -> (deleted portion=w5284:bool[], array with subset deleted=w5267:bool[])
                n3642 = Index Array(array=w5294, index #1=5 ("索引"), index #2=6 ("索引")) -> (element #1=w5283:bool, element #2=w5266:bool)
                n3643 = Index Array(array=w5286) -> (element #1=w5279:bool, element #2=w5262:bool)  [unwired: 2 in]
                n3644 = Array Subset(array=w5272, index=2 ("索引"), length=3 ("长度")) -> (w5281:bool[])
                n3645 = Delete From Array(array=w5271, length=3 ("索引"), index=2 ("长度")) -> (deleted portion=w5282:bool[], array with subset deleted=w5265:bool[])
                n3646 = Array Subset(array=w5275, index=4 ("索引"), length=2 ("长度")) -> (w5280:bool[])
                n3647 = Delete From Array(array=w5301, index=w5300) -> (deleted portion=w5298:refnum<vi>, array with subset deleted=w5299:refnum<vi>[])  [unwired: 1 in]
                n3648 = Insert Into Array(array=w5285, new element #1=w5284, new element #2=w5283, new element #3=w5282, new element #4=w5281, new element #5=w5280, new element #6=w5279) -> (w5278:bool[])  [unwired: 1 in]
                n3649 = Array Subset(array=w5275, index=6 ("索引"), length=2 ("长度")) -> (w5263:bool[])
                n3650 = Array Subset(array=w5272, index=5 ("索引"), length=3 ("长度")) -> (w5264:bool[])
                n3651 = And Array Elements(Boolean array=w5278) -> (logical AND=w5260:bool)
                n3652 = Insert Into Array(array=w5267, new element #1=w5266, new element #2=w5265, new element #3=w5264, new element #4=w5263, new element #5=w5262) -> (w5261:bool[])  [unwired: 1 in]
                n3653 = And Array Elements(Boolean array=w5261) -> (logical AND=w5259:bool)
              }
              frame "单选选项2" {
                n3654 = global read "功能码全局.vi" "18"() -> (w5316:bool[])
                n3655 = global read "功能码全局.vi" "15"() -> (w5337:bool[])
                n3656 = global read "功能码全局.vi" "16"() -> (w5334:bool[])
                n3657 = Delete From Array(array=w5342, index=w5343) -> (deleted portion=w5340:refnum<vi>, array with subset deleted=w5341:refnum<vi>[])  [unwired: 1 in]
                n3658 = Index Array(array=w5334, index #1=4 ("索引"), index #2=5 ("索引"), index #3=6 ("索引"), index #4=7 ("索引")) -> (element #1=w5328:bool, element #2=w5327:bool, element #3=w5323:bool, element #4=w5322:bool)
                n3659 = Index Array(array=w5316, index #1=4 ("索引"), index #2=5 ("索引"), index #3=6 ("索引"), index #4=7 ("索引"), index #5=2 ("索引"), index #6=3 ("索引"), index #7=0 ("索引"), index #8=1 ("索引")) -> (element #1=w5309:bool, element #2=w5312:bool, element #3=w5311:bool, element #4=w5310:bool, element #5=w5308:bool, element #6=w5307:bool, element #7=w5302:bool, element #8=w5303:bool)
                n3660 = Delete From Array(array=w5337, length=4 ("长度"), index=0 ("索引")) -> (deleted portion=w5329:bool[], array with subset deleted=w5324:bool[])
                n3661 = Insert Into Array(array=w5324, new element #1=w5323, new element #2=w5322, new element #3=w5312, new element #4=w5311, new element #5=w5310, new element #6=w5303) -> (w5321:bool[])  [unwired: 1 in]
                n3662 = Insert Into Array(array=w5329, new element #1=w5328, new element #2=w5327, new element #3=w5309, new element #4=w5308, new element #5=w5307, new element #6=w5302) -> (w5326:bool[])  [unwired: 1 in]
                n3663 = And Array Elements(Boolean array=w5326) -> (logical AND=w5325:bool)
                n3664 = And Array Elements(Boolean array=w5321) -> (logical AND=w5320:bool)
              }
            }
            n3665 = property on="全部写入" class="Bool (严格)"("Visible"=w5242) -> ()  [unwired: 2 in, 2 out]
            n3666 = property on="全部读取" class="Bool (严格)"("Visible"=w5241) -> ()  [unwired: 2 in, 2 out]
            n3667 = property on="从板号" class="DigNum (严格)"("Visible"=w5239) -> ()  [unwired: 2 in, 2 out]
            n3668 = local write "主从选择"(w5253) -> ()
            n3669 = property on="从板个数" class="DigNum (严格)"("Visible"=w5245) -> ()  [unwired: 2 in, 2 out]
            n3670 = for {
              tunnel: u32 87470 -> [w5257]
              tunnel: w5250 -> [w5256] mode=indexing
              n3671 = property class="Bool (严格)"(reference=w5256, "BoolText.TextColor"=w5257) -> ()  [unwired: 1 in, 2 out]
            }
            n3672 = Not(x=w5245) -> (.not. x?=w5246:bool)
            n3673 = property class="Bool (严格)"(reference=w5249, "BoolText.TextColor"=u32 16777215) -> ()  [unwired: 1 in, 2 out]
            n3674 = property on="主板选项" class="Tree (严格)"("Visible"=w5245) -> ()  [unwired: 2 in, 2 out]
            n3675 = property on="从板选项" class="Tree (严格)"("Visible"=w5246) -> ()  [unwired: 2 in, 2 out]
            n3676 = property on="当前从板板号" class="DigNum (严格)"("Visible"=w5246) -> ()  [unwired: 2 in, 2 out]
            n3677 = property on="单个读取" class="Bool (严格)"("Visible"=w5240) -> ()  [unwired: 2 in, 2 out]
            n3678 = property on="单个写入" class="Bool (严格)"("Visible"=w5240) -> ()  [unwired: 2 in, 2 out]
          }
          event "从板号": Value Change {
            n3679 = event-data() -> ()  [unwired: 7 out]
            n3680 = local read "key names"() -> (w5345:string[])
            n3681 = Empty Array?(array=w5345) -> (empty?=w5344:bool)
            n3682 = case shown="假" w5344 {
              tunnel: w5345 -> [w5348 _]
              frame False {
                n3683 = stacked-sequence {
                  seq-local: [w5349 _] -> [_ w5412]
                  tunnel: w5348 -> [w5357 _]
                  frame #0 {
                    w5388 = 2 ("长度")
                    w5385 = 20 ("长度")
                    w5373 = 1 ("索引")
                    n3684 = local read "从板号"() -> (w5349:u8)
                    n3685 = local read "输出数组"() -> (w5358:string[][])
                    n3686 = Decrement(x=w5349) -> (x-1=w5355:u8)
                    n3687 = Index Array(array=w5358, index (col)=w5355) -> (element=w5386:string[])  [unwired: 1 in]
                    n3688 = global write "读配置文件全局2.vi" "从板板号"(w5349) -> ()
                    n3689 = Search 1D Array(1D array=w5357, element="风机开启温度" ("元素")) -> (index of element=w5370:i32)  [unwired: 1 in]
                    n3690 = Search 1D Array(1D array=w5357, element="电压过高一级" ("元素"), start index (0)=w5370) -> (index of element=w5368:i32)
                    n3691 = Decrement(x=w5370) -> (x-1=w5372:i32)
                    n3692 = Array Subset(array=w5386, index=w5373, length=w5372) -> (w5356:string[])
                    n3693 = Array Subset(array=w5386, index=w5368, length=21 ("长度")) -> (w5360:string[])
                    n3694 = Array Subset(array=w5357, index=w5373, length=w5372) -> (w5403:string[])
                    n3695 = Array Subset(array=w5386, index=w5370, length=7 ("长度")) -> (w5366:string[])
                    n3696 = for {
                      tunnel: w5360 -> [w5405] mode=indexing
                      tunnel: [w5404] -> w5359 mode=indexing
                      n3697 = Fract/Exp String To Number(string=w5405) -> (number=w5404:dbl)  [unwired: 3 in, 1 out]
                    }
                    n3698 = for {
                      tunnel: w5366 -> [w5407] mode=indexing
                      tunnel: [w5406] -> w5350 mode=indexing
                      n3699 = Fract/Exp String To Number(string=w5407) -> (number=w5406:dbl)  [unwired: 3 in, 1 out]
                    }
                    n3700 = Delete From Array(array=w5359, length=7 ("长度"), index=0 ("索引")) -> (deleted portion=w5353:dbl[], array with subset deleted=w5363:dbl[])
                    n3701 = Array To Cluster(array=w5350) -> (cluster=w5375:T27)
                    n3702 = global write "读配置文件全局2.vi" "加热控制参数"(w5350) -> ()
                    n3703 = Delete From Array(array=w5363, length=7 ("长度"), index=0 ("索引")) -> (deleted portion=w5352:dbl[], array with subset deleted=w5351:dbl[])
                    n3704 = local write "加热控制参数"(w5375) -> ()
                    n3705 = Array To Cluster(array=w5353) -> (cluster=w5400:T27)
                    n3706 = Array To Cluster(array=w5351) -> (cluster=w5402:T27)
                    n3707 = Array To Cluster(array=w5352) -> (cluster=w5401:T27)
                    n3708 = global write "读配置文件全局2.vi" "三级故障阀值"(w5351) -> ()
                    n3709 = global write "读配置文件全局2.vi" "一级故障阀值"(w5353) -> ()
                    n3710 = global write "读配置文件全局2.vi" "二级故障阀值"(w5352) -> ()
                    n3711 = local write "一级故障 6"(w5400) -> ()
                    n3712 = local write "一级故障 8"(w5402) -> ()
                    n3713 = local write "一级故障 7"(w5401) -> ()
                    n3714 = Search 1D Array(1D array=w5403, element="温度个数" ("元素")) -> (index of element=w5382:i32)  [unwired: 1 in]
                    n3715 = Search 1D Array(1D array=w5403, element="第一个保险通道" ("元素")) -> (index of element=w5383:i32)  [unwired: 1 in]
                    n3716 = Search 1D Array(1D array=w5403, element="电压个数" ("元素")) -> (index of element=w5381:i32)  [unwired: 1 in]
                    n3717 = Search 1D Array(1D array=w5403, element="第1通道电压个数" ("元素")) -> (index of element=w5384:i32)  [unwired: 1 in]
                    n3718 = Array Subset(array=w5356, index=w5381, length=2 ("长度")) -> (w5389:string[])
                    n3719 = Array Subset(array=w5356, index=w5382, length=w5388) -> (w5391:string[])
                    n3720 = Array Subset(array=w5356, index=w5383, length=20 ("长度")) -> (w5392:string[])
                    n3721 = Array Subset(array=w5356, index=w5384, length=w5385) -> (w5390:string[])
                    n3722 = Insert Into Array(array=w5389, new element #1=w5390, new element #2=w5391, new element #3=w5392) -> (w5354:string[])  [unwired: 1 in]
                    n3723 = Array Subset(array=w5403, index=w5381, length=w5388) -> (w5393:string[])
                    n3724 = Array Subset(array=w5403, index=w5382, length=w5388) -> (w5395:string[])
                    n3725 = Array Subset(array=w5403, index=w5383, length=w5385) -> (w5396:string[])
                    n3726 = Array Subset(array=w5403, index=w5384, length=w5385) -> (w5394:string[])
                    n3727 = global write "读配置文件全局2.vi" "表格"(w5354) -> ()
                    n3728 = Insert Into Array(array=w5393, new element #1=w5394, new element #2=w5395, new element #3=w5396) -> (w5398:string[])  [unwired: 1 in]
                    n3729 = Build Array(w5398, w5354) -> (w5397:string[][])
                    n3730 = Transpose 2D Array(2D array=w5397) -> (transposed array=w5399:string[][])
                    n3731 = local write "项目信息 2"(w5399) -> ()
                  }
                  frame #1 {
                    n3732 = Number To Decimal String(number=w5412) -> (decimal integer string=w5410:string)  [unwired: 1 in]
                    n3733 = control-ref of="结果"() -> (w5415:refnum<vi>)
                    n3734 = Concatenate Strings("从板", w5410, "导入完成") -> (w5408:string)
                    n3735 = Build Array(w5408) -> (w5413:string[])
                    n3736 = call "表格编辑.vi"("新元素/子数组"=w5413, "活动单元格:单元格背景色"=u32 6618880, "MCListbox引用句柄"=w5415) -> ()  [unwired: 9 out]
                  }
                }
              }
              frame True {
              }
            }
          }
